vi "Read Connection Ref.vi"(8 "error in (no error)":errorcluster, 11 "Agilent 34401A in":refnum<class "Agilent 34401A.lvclass">) -> (0 "error out":errorcluster, 2 "Connection Ref":variant, 3 "Agilent 34401A out":refnum<class "Agilent 34401A.lvclass">)   [LabVIEW 2021, in "DMM.lvlib" / "Agilent 34401A.lvclass"]
uses:
  Agilent 34401A.lvclass
  Agilent 34401A.lvclass/Agilent 34401A.ctl
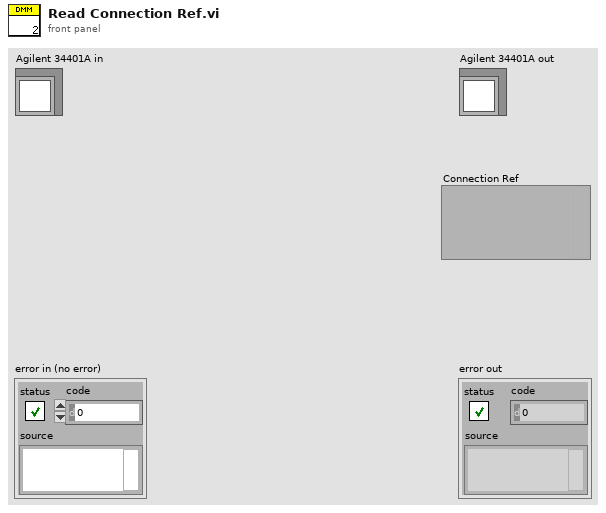
[diagram p1: front panel]
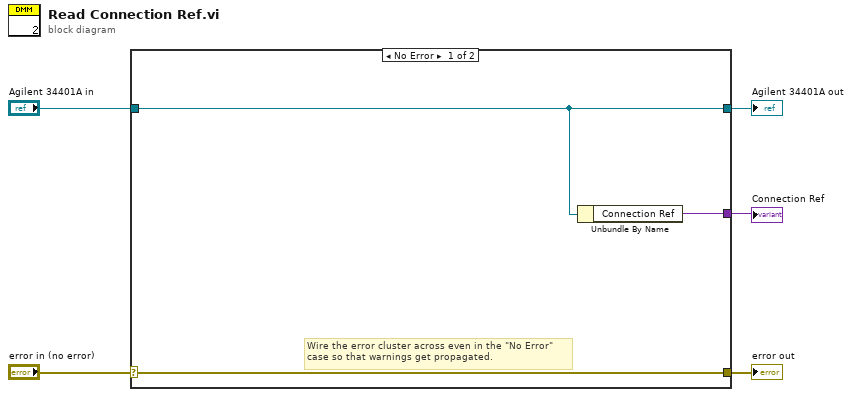
[diagram p0: block diagram]
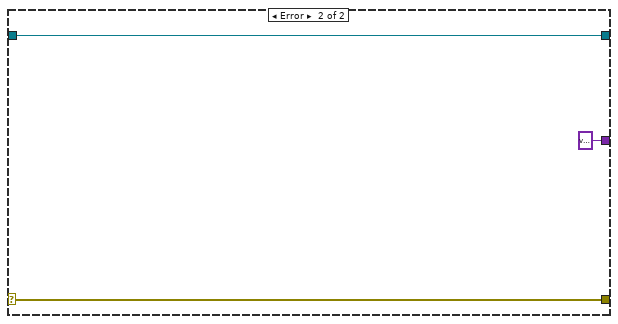
[diagram p2: hidden frame]
diagram:
  n1 = case shown="No Error" "error in (no error)" {
    selector: "error in (no error)" -> [w8 w11]
    tunnel: [w8 w11] -> w4
    tunnel: [w7 w10] -> w2
    tunnel: "Agilent 34401A in" -> [w7 w10]
    tunnel: [w6 variant ("Connection Ref")] -> w1
    frame No Error {
      # "Wire the error cluster across even in the \"No Error\"\ncase so that warnings get propagated."
      n2 = Unbundle By Name(w7) -> ("Connection Ref"=w6:variant)
    }
    frame Error {
    }
  }
  "error out" <- w4
  "Agilent 34401A out" <- w2
  "Connection Ref" <- w1
